vi "Read previous_state.vi"(8 "error in (no error)":errorcluster, 11 "State Machine in":refnum<class "State Machine.lvclass">) -> (0 "error out":errorcluster, 2 "previous_state":u32, 3 "State Machine out":refnum<class "State Machine.lvclass">)   [LabVIEW 2018, in "State Machine.lvclass"]
doc: "Este VI faz a leitura do estado anterior."
uses:
  State Machine.lvclass
  State Machine.lvclass/State Machine.ctl
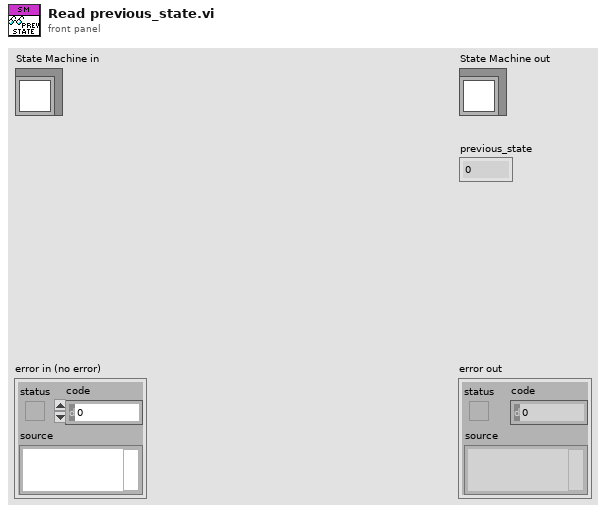
[diagram p1: front panel]
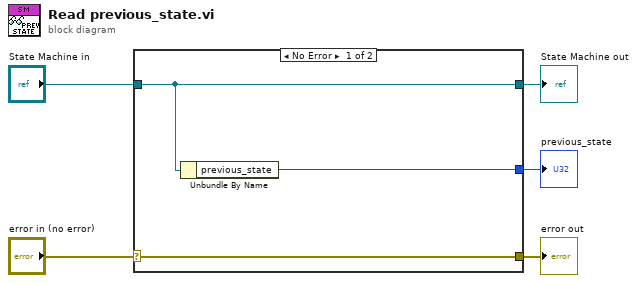
[diagram p0: block diagram]
diagram:
  n1 = case shown="No Error" "error in (no error)" {
    selector: "error in (no error)" -> [w8 w9]
    tunnel: [w8 w9] -> w4
    tunnel: [w7 w10] -> w2
    tunnel: "State Machine in" -> [w7 w10]
    tunnel: [w6 _] -> w1
    frame No Error {
      n2 = Unbundle By Name(w7) -> ("previous_state"=w6:u32)
    }
    frame Error {
    }
  }
  "error out" <- w4
  "State Machine out" <- w2
  "previous_state" <- w1
